vi "Format View Parameter.vi"(8 "error in (no error)":errorcluster, 10 "Column":T1, 11 "VI in":refnum<class "VI.lvclass">) -> (0 "error out":errorcluster, 2 "View Parameter":string, 3 "VI out":refnum<class "VI.lvclass">)   [LabVIEW 2020, in "VI Properties Editor.lvlib" / "VI.lvclass"]
doc: "Formats a parameter to sort by, based on <B>Column</B>."
uses:
  VI.lvclass
  C:/Users/acasalen/Documents/LabVIEW Data/Projects/VI-Properties-Editor/source/Classes/Item/Item.lvclass
  CTLs/Sort Column.ctl
  VI Properties Editor.lvlib
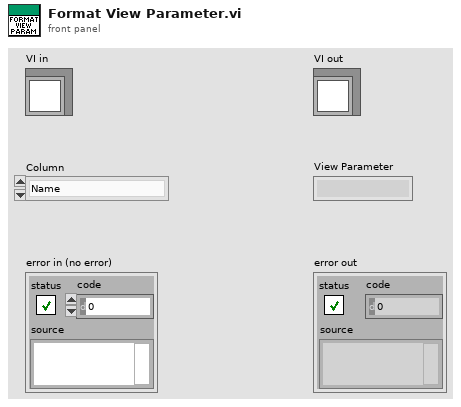
[diagram p1: front panel]
types:
  T1 = typedef "VI Properties Editor.lvlib/Sort Column.ctl" = enum16{"Name", "Filename", "Path", "Type", "Window Title", "Description", "Help Path", "Help Tag", "Custom Title?", "Reentrancy", "Inlined?", "Help URL", "Help Type", "Allow Debugging?", "Auto Error Handling?", "Run When Opened?", "Suspend When Called?", "Priority", "Preferred Exec Sytem"}
  T2 = enum32{"invalid VI type", "Standard VI", "Control VI", "Global VI", "Polymorphic VI", "Configuration VI", "SubSystem", "Facade VI", "Method VI", "Statechart Diagram VI"}
  T3 = enum16{"Share clones between instances", "Preallocate clone for each instance"}
  T4 = enum32{"invalid priority", "background priority", "normal priority", "above normal priority", "high priority", "time critical priority", "subroutine"}
  T5 = enum32{"invalid execution system", "user interface", "standard", "instrument i/o", "data acquisition", "other 1", "other 2", "same as caller"}
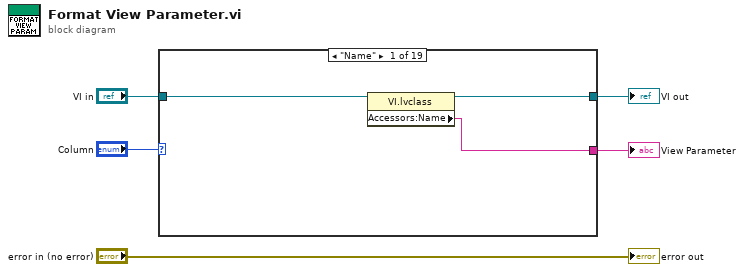
[diagram p0: block diagram]
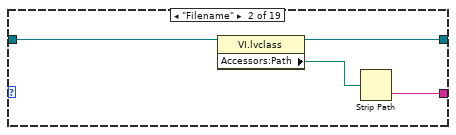
[diagram p2: hidden frame]
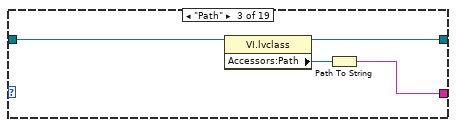
[diagram p3: hidden frame]
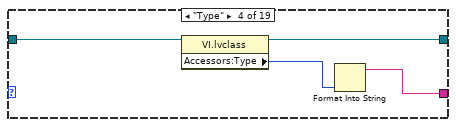
[diagram p4: hidden frame]
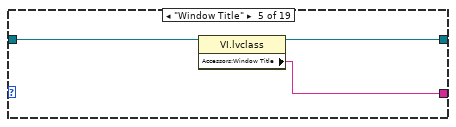
[diagram p5: hidden frame]
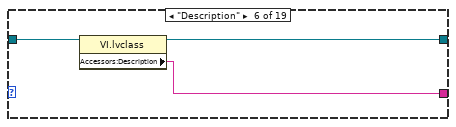
[diagram p6: hidden frame]
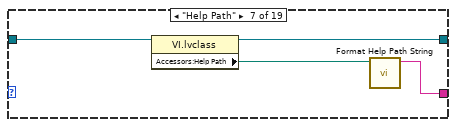
[diagram p7: hidden frame]
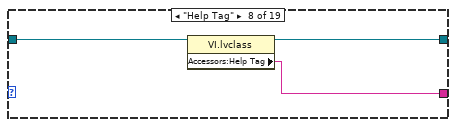
[diagram p8: hidden frame]
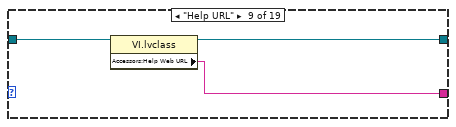
[diagram p9: hidden frame]
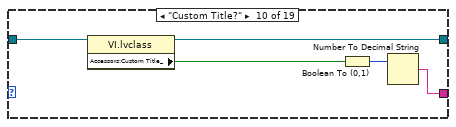
[diagram p10: hidden frame]
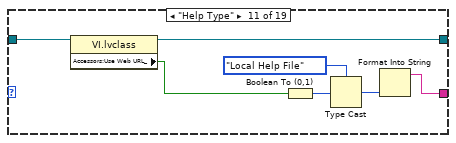
[diagram p11: hidden frame]
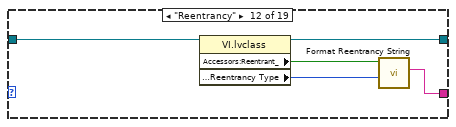
[diagram p12: hidden frame]
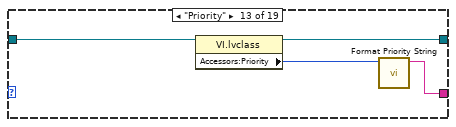
[diagram p13: hidden frame]
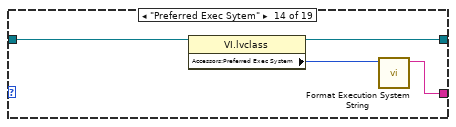
[diagram p14: hidden frame]
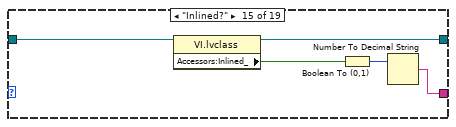
[diagram p15: hidden frame]
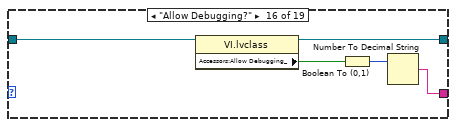
[diagram p16: hidden frame]
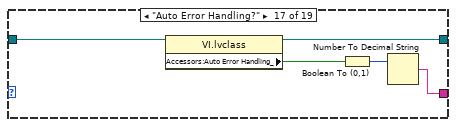
[diagram p17: hidden frame]
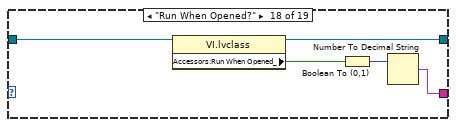
[diagram p18: hidden frame]
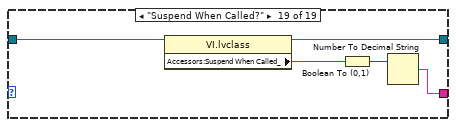
[diagram p19: hidden frame]
diagram:
  n1 = case shown="\"Name\"" "Column" {
    tunnel: [w6 w9 w16 w20 w21 w24 w30 w31 w34 w40 w45 w53 w57 w61 w65 w70 w75 w80 w85] -> w1
    tunnel: "VI in" -> [w8 w12 w15 w19 w23 w26 w29 w33 w36 w39 w44 w52 w56 w60 w64 w69 w74 w79 w84]
    tunnel: [w7 w11 w14 w18 w22 w25 w27 w32 w35 w38 w42 w49 w55 w59 w63 w68 w72 w77 w83] -> w2
    frame "Name" {
      n2 = property class="VI.lvclass"(reference=w8) -> (reference out=w7:refnum<class "VI.lvclass">, "Accessors:Name"=w6:string)  [unwired: 1 in, 1 out]
    }
    frame "Filename" {
      n3 = property class="VI.lvclass"(reference=w12) -> (reference out=w11:refnum<class "VI.lvclass">, "Accessors:Path"=w10:path)  [unwired: 1 in, 1 out]
      n4 = Strip Path(path=w10) -> (name=w9:string)  [unwired: 1 out]
    }
    frame "Path" {
      n5 = property class="VI.lvclass"(reference=w15) -> (reference out=w14:refnum<class "VI.lvclass">, "Accessors:Path"=w13:path)  [unwired: 1 in, 1 out]
      n6 = Path To String(path=w13) -> (string=w16:string)
    }
    frame "Type" {
      n7 = property class="VI.lvclass"(reference=w19) -> (reference out=w18:refnum<class "VI.lvclass">, "Accessors:Type"=w17:T2)  [unwired: 1 in, 1 out]
      n8 = Format Into String(w17) -> (resulting string=w20:string)  [unwired: 3 in, 1 out]
    }
    frame "Window Title" {
      n9 = property class="VI.lvclass"(reference=w23) -> (reference out=w22:refnum<class "VI.lvclass">, "Accessors:Window Title"=w21:string)  [unwired: 1 in, 1 out]
    }
    frame "Description" {
      n10 = property class="VI.lvclass"(reference=w26) -> (reference out=w25:refnum<class "VI.lvclass">, "Accessors:Description"=w24:string)  [unwired: 1 in, 1 out]
    }
    frame "Help Path" {
      n11 = property class="VI.lvclass"(reference=w29) -> (reference out=w27:refnum<class "VI.lvclass">, "Accessors:Help Path"=w28:path)  [unwired: 1 in, 1 out]
      n12 = call "Format Help Path String.vi"("Help Path"=w28) -> ("Help Path String"=w30:string)  [unwired: 10 in]
    }
    frame "Help Tag" {
      n13 = property class="VI.lvclass"(reference=w33) -> (reference out=w32:refnum<class "VI.lvclass">, "Accessors:Help Tag"=w31:string)  [unwired: 1 in, 1 out]
    }
    frame "Help URL" {
      n14 = property class="VI.lvclass"(reference=w36) -> (reference out=w35:refnum<class "VI.lvclass">, "Accessors:Help Web URL"=w34:string)  [unwired: 1 in, 1 out]
    }
    frame "Custom Title?" {
      n15 = property class="VI.lvclass"(reference=w39) -> (reference out=w38:refnum<class "VI.lvclass">, "Accessors:Custom Title_"=w37:bool)  [unwired: 1 in, 1 out]
      n16 = Boolean To (0,1)(Boolean=w37) -> (0, 1=w41:i16)
      n17 = Number To Decimal String(number=w41) -> (decimal integer string=w40:string)  [unwired: 1 in]
    }
    frame "Help Type" {
      n18 = property class="VI.lvclass"(reference=w44) -> (reference out=w42:refnum<class "VI.lvclass">, "Accessors:Use Web URL_"=w43:bool)  [unwired: 1 in, 1 out]
      n19 = Boolean To (0,1)(Boolean=w43) -> (0, 1=w48:i16)
      n20 = Type Cast(type=enum16{"Local Help File", "Web-based Help"}."Local Help File" ("FP.Help Type"), x=w48) -> (*(type *) &x=w46:enum16{"Local Help File", "Web-based Help"})
      n21 = Format Into String(w46) -> (resulting string=w45:string)  [unwired: 3 in, 1 out]
    }
    frame "Reentrancy" {
      n22 = property class="VI.lvclass"(reference=w52) -> (reference out=w49:refnum<class "VI.lvclass">, "Accessors:Reentrant_"=w51:bool, "Accessors:Reentrancy Type"=w50:T3)  [unwired: 1 in, 1 out]
      n23 = call "Format Reentrancy String.vi"("Reentrancy Type"=w50, "Reentrant?"=w51) -> ("Reentrancy String"=w53:string)  [unwired: 9 in]
    }
    frame "Priority" {
      n24 = property class="VI.lvclass"(reference=w56) -> (reference out=w55:refnum<class "VI.lvclass">, "Accessors:Priority"=w54:T4)  [unwired: 1 in, 1 out]
      n25 = call "Format Priority String.vi"("Priority"=w54) -> ("Priority String"=w57:string)  [unwired: 10 in]
    }
    frame "Preferred Exec Sytem" {
      n26 = property class="VI.lvclass"(reference=w60) -> (reference out=w59:refnum<class "VI.lvclass">, "Accessors:Preferred Exec System"=w58:T5)  [unwired: 1 in, 1 out]
      n27 = call "Format Execution System String.vi"("Preferred Exec System"=w58) -> ("Preferred Exec System String"=w61:string)  [unwired: 10 in]
    }
    frame "Inlined?" {
      n28 = property class="VI.lvclass"(reference=w64) -> (reference out=w63:refnum<class "VI.lvclass">, "Accessors:Inlined_"=w62:bool)  [unwired: 1 in, 1 out]
      n29 = Boolean To (0,1)(Boolean=w62) -> (0, 1=w66:i16)
      n30 = Number To Decimal String(number=w66) -> (decimal integer string=w65:string)  [unwired: 1 in]
    }
    frame "Allow Debugging?" {
      n31 = property class="VI.lvclass"(reference=w69) -> (reference out=w68:refnum<class "VI.lvclass">, "Accessors:Allow Debugging_"=w67:bool)  [unwired: 1 in, 1 out]
      n32 = Boolean To (0,1)(Boolean=w67) -> (0, 1=w71:i16)
      n33 = Number To Decimal String(number=w71) -> (decimal integer string=w70:string)  [unwired: 1 in]
    }
    frame "Auto Error Handling?" {
      n34 = property class="VI.lvclass"(reference=w74) -> (reference out=w72:refnum<class "VI.lvclass">, "Accessors:Auto Error Handling_"=w73:bool)  [unwired: 1 in, 1 out]
      n35 = Boolean To (0,1)(Boolean=w73) -> (0, 1=w76:i16)
      n36 = Number To Decimal String(number=w76) -> (decimal integer string=w75:string)  [unwired: 1 in]
    }
    frame "Run When Opened?" {
      n37 = property class="VI.lvclass"(reference=w79) -> (reference out=w77:refnum<class "VI.lvclass">, "Accessors:Run When Opened_"=w78:bool)  [unwired: 1 in, 1 out]
      n38 = Boolean To (0,1)(Boolean=w78) -> (0, 1=w81:i16)
      n39 = Number To Decimal String(number=w81) -> (decimal integer string=w80:string)  [unwired: 1 in]
    }
    frame "Suspend When Called?" {
      n40 = property class="VI.lvclass"(reference=w84) -> (reference out=w83:refnum<class "VI.lvclass">, "Accessors:Suspend When Called_"=w82:bool)  [unwired: 1 in, 1 out]
      n41 = Boolean To (0,1)(Boolean=w82) -> (0, 1=w86:i16)
      n42 = Number To Decimal String(number=w86) -> (decimal integer string=w85:string)  [unwired: 1 in]
    }
  }
  "VI out" <- w2
  "View Parameter" <- w1
  "error out" <- "error in (no error)"
